vi "Update BuildSpecs.vi"(8 "error in (no error)":errorcluster, 11 "CD Build Tools in":refnum<class "Project Sync Tools.lvclass">) -> (0 "error out":errorcluster, 3 "CD Build Tools out":refnum<class "Project Sync Tools.lvclass">)   [LabVIEW 2019, in "Project Sync Tools.lvclass"]
uses:
  Project Sync Tools.lvclass
  Project Sync Tools.lvclass/Project Sync Tools.ctl
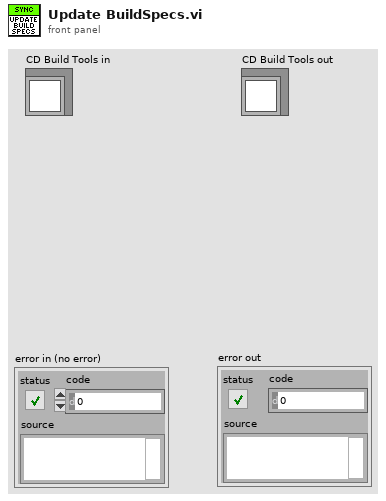
[diagram p1: front panel]
types:
  T1 = typedef "Project Sync Tools.lvclass/BuildSpec Parameters.ctl" = cluster{"BuildSpec Ref":refnum<vi>, "Target Name":string, "Build Spec Name":string, "Tags":string[], "Tag Values":variant[]}
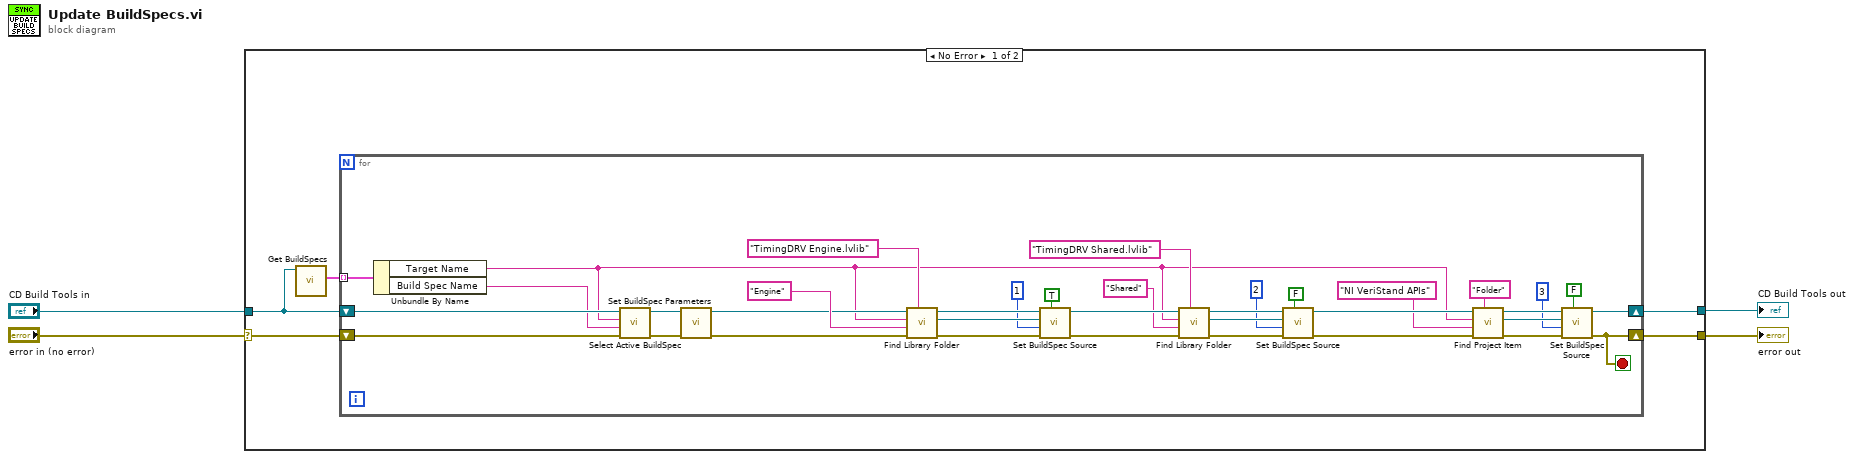
[diagram p0: block diagram]
diagram:
  n1 = case shown="No Error" "error in (no error)" {
    selector: "error in (no error)" -> [w7 w47]
    tunnel: "CD Build Tools in" -> [w8 w46]
    tunnel: [w6 w46] -> w3
    tunnel: [w5 w47] -> w1
    frame No Error {
      n2 = call "Get BuildSpecs.vi"("Project Sync Tools in"=w8) -> ("BuildSpecs"=w9:T1[])  [unwired: 9 in, 1 out]
      n3 = for {
        shift-right: [w10] -> w5
        shift-left: w7 -> [w43]
        shift-right: [w15] -> w6
        shift-left: w8 -> [w14]
        tunnel: w9 -> [w13] mode=indexing
        stop <- w10 stop-if-true
        n4 = Unbundle By Name(w13) -> ("Target Name"=w12:string, "Build Spec Name"=w11:string)
        n5 = call "Select Active BuildSpec.vi"("error in (no error)"=w43, "Build Spec Name in"=w11, "Target Name in"=w12, "Project Sync Tools in"=w14) -> ("error out"=w42:errorcluster, "Project Sync Tools out"=w41:refnum<class "Project Sync Tools.lvclass">)  [unwired: 6 in]
        n6 = call "Set BuildSpec Parameters.vi"("Error In"=w42, "Project Sync Tools in"=w41) -> ("error out"=w40:errorcluster, "Project Sync Tools out"=w39:refnum<class "Project Sync Tools.lvclass">)  [unwired: 8 in]
        n7 = call "Find Library Folder.vi"("Library Name"="TimingDRV Engine.lvlib", "error in (no error)"=w40, "Folder Name"="Engine" ("Target Item Name"), "Target Name"=w12, "Project Sync Tools in"=w39) -> ("error out"=w38:errorcluster, "Folder Ref out"=w37:refnum<vi>, "Project Sync Tools out"=w36:refnum<class "Project Sync Tools.lvclass">)  [unwired: 3 in, 1 out]
        n8 = call "Set BuildSpec Source.vi"("Apply Inclusion ?"=TRUE, "Error In"=w38, "Source Index"=1, "Source Item in"=w37, "Project Sync Tools in"=w36) -> ("error out"=w31:errorcluster, "Project Sync Tools out"=w33:refnum<class "Project Sync Tools.lvclass">)  [unwired: 5 in]
        n9 = call "Find Library Folder.vi"("Library Name"="TimingDRV Shared.lvlib", "error in (no error)"=w31, "Folder Name"="Shared", "Target Name"=w12, "Project Sync Tools in"=w33) -> ("error out"=w29:errorcluster, "Folder Ref out"=w27:refnum<vi>, "Project Sync Tools out"=w28:refnum<class "Project Sync Tools.lvclass">)  [unwired: 3 in, 1 out]
        n10 = call "Set BuildSpec Source.vi"("Apply Inclusion ?"=FALSE, "Error In"=w29, "Source Index"=2, "Source Item in"=w27, "Project Sync Tools in"=w28) -> ("error out"=w24:errorcluster, "Project Sync Tools out"=w23:refnum<class "Project Sync Tools.lvclass">)  [unwired: 5 in]
        n11 = call "Find Project Item.vi"("Type"="Folder", "error in (no error)"=w24, "Item Name"="NI VeriStand APIs", "Target Name"=w12, "Project Sync Tools in"=w23) -> ("error out"=w20:errorcluster, "ProjectItem out"=w18:refnum<vi>, "Project Sync Tools out"=w19:refnum<class "Project Sync Tools.lvclass">)  [unwired: 3 in, 1 out]
        n12 = call "Set BuildSpec Source.vi"("Apply Inclusion ?"=FALSE, "Error In"=w20, "Source Index"=3, "Source Item in"=w18, "Project Sync Tools in"=w19) -> ("error out"=w10:errorcluster, "Project Sync Tools out"=w15:refnum<class "Project Sync Tools.lvclass">)  [unwired: 5 in]
      }
    }
    frame Error {
    }
  }
  "CD Build Tools out" <- w3
  "error out" <- w1
